vi "BIN-filenum2daynum.vi"(2 "FileNum":u64) -> (7 "DayNum":u64)   [LabVIEW 2020]
doc: "Convert date to YYYYMMDD numerical value"
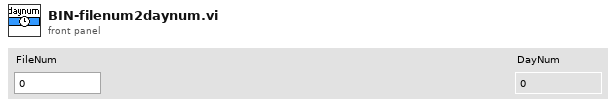
[diagram p1: front panel]
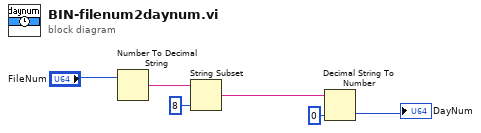
[diagram p0: block diagram]
diagram:
  n1 = Number To Decimal String(number="FileNum") -> (decimal integer string=w3:string)  [unwired: 1 in]
  n2 = String Subset(string=w3, length (rest)=8 ("length (rest)")) -> (substring=w1:string)  [unwired: 1 in]
  n3 = Decimal String To Number(string=w1, default (0L)=u64 0 ("default (0 I32)")) -> (number=→"DayNum":u64)  [unwired: 1 in, 1 out]
